vi "Can接收.vi"(7 "CANPort":u16, 9 "匹配CANID":u32 format="%x") -> (0 "接收数据":u8[](array[numeric]), 2 "成功？":bool)   [LabVIEW 2010]
uses:
  全局量/全局_配置.vi
panel:
  out "开始时间":dbl format="%#.0f"
  in  "Baudrate":u32(ring)=1000 caption="K" items=["10"=10, "20"=20, "50"=50, "100"=100, "125"=125, "250"=250, "500"=500, "800"=800, "250"=1000]
  out "Error out":errorcluster {"code" format="%.0x"}
  in  "ReadTimeOut":u32=3000 caption="ms"
  in  "Synchronization":i32(ring)=1 items=["Synchronization"=1, "Asynchronization"=0]
  # "从1开始"
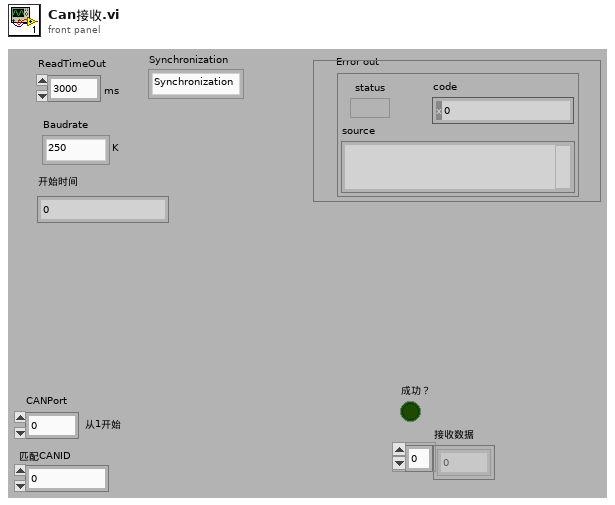
[diagram p1: front panel]
types:
  T1 = cluster{"Internal":u32, "InternalHigh":u32, "Offset":u32, "OffsetHigh":u32, "hEvent":u32}
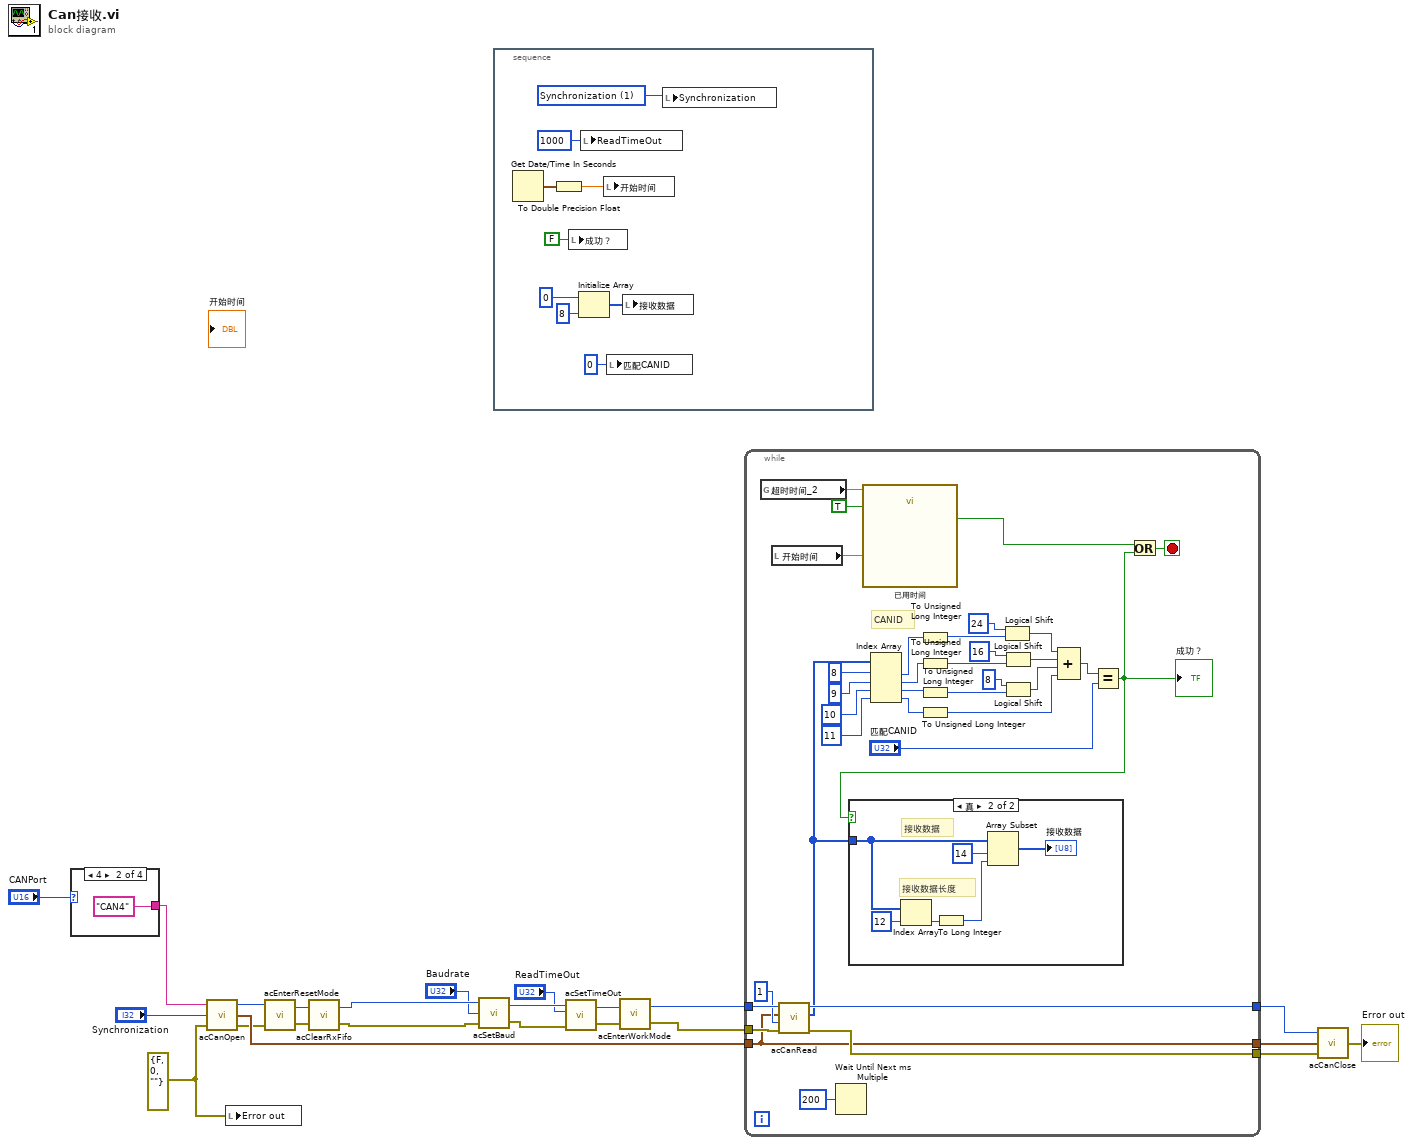
[diagram p0: block diagram]
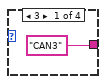
[diagram p3: hidden frame]
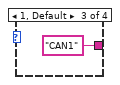
[diagram p4: hidden frame]
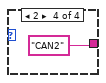
[diagram p5: hidden frame]
diagram:
  w17 = errorcluster {"status"=FALSE, "code"=0, "source"=""} ("Error in")
  n1 = case shown="4" "CANPort" {
    tunnel: ["CAN3" "CAN4" "CAN1" "CAN2"] -> w2
    frame 3 {
    }
    frame 4 {
    }
    frame 1, Default {
    }
    frame 2 {
    }
  }
  n2 = call "acCanOpen.vi"("Error in"=w17, "Synchronization"="Synchronization", "CANPort"=w2) -> ("Error out"=w18:errorcluster, "Overlapped"=w21:T1, "Handle"=w19:u32)
  n3 = local write "Error out"(w17) -> ()
  n4 = call "acEnterResetMode.vi"("Error in"=w18, "Handle  in"=w19) -> ("Error out"=w12:errorcluster, "Handle out"=w11:u32)
  n5 = call "acClearRxFifo.vi"("Error in"=w12, "Handle  in"=w11) -> ("Error out"=w9:errorcluster, "Handle out"=w10:u32)
  n6 = call "acSetBaud.vi"("Error in"=w9, "Baudrate"="Baudrate", "Handle  in"=w10) -> ("Error out"=w14:errorcluster, "Handle out"=w15:u32)
  n7 = stacked-sequence {
    frame #0 {
      w34 = 1 items=["Synchronization"=1, "Asynchronization"=0] ("Synchronization")
      n8 = Get Date/Time In Seconds() -> (seconds since 1Jan1904=w30:timestamp)
      n9 = To Double Precision Float(number=w30) -> (double precision float=w29:dbl)
      n10 = local write "成功？"(FALSE ("成功？")) -> ()
      n11 = Initialize Array(u8 0, 8 ("维数大小")) -> (w31:u8[])
      n12 = local write "ReadTimeOut"(u32 1000 ("ReadTimeOut")) -> ()
      n13 = local write "开始时间"(w29) -> ()
      n14 = local write "匹配CANID"(u32 0 ("匹配CANID")) -> ()
      n15 = local write "接收数据"(w31) -> ()
      n16 = local write "Synchronization"(w34) -> ()
    }
  }
  n17 = call "acSetTimeOut.vi"("Error in"=w14, "Read TimeOut"="ReadTimeOut", "Handle  in"=w15) -> ("Error out"=w7:errorcluster, "Handle out"=w8:u32)  [unwired: 1 in]
  n18 = call "acEnterWorkMode.vi"("Error in"=w7, "Handle  in"=w8) -> ("Error out"=w5:errorcluster, "Handle out"=w6:u32)
  n19 = while {
    tunnel: [w70] -> w22
    tunnel: w21 -> [w65]
    tunnel: [w69] -> w20
    tunnel: w6 -> [w68]
    tunnel: w5 -> [w67]
    tunnel: [w65] -> w1
    stop <- w60 stop-if-true
    # "CANID"
    n20 = global read "全局_配置.vi" "超时时间_2"() -> (w63:dbl)
    n21 = local read "开始时间"() -> (w62:dbl)
    n22 = call "acCanRead.vi"("Error in"=w67, "ReadCount"=u32 1 ("接收CAN帧数 2"), "Overlapped"=w65, "Handle  in"=w68) -> ("Error out"=w69:errorcluster, "MSG"=w38:u8[], "Handle out"=w70:u32)  [unwired: 1 out]
    n23 = Wait Until Next ms Multiple(millisecond multiple=u32 200 ("毫秒倍数")) -> ()  [unwired: 1 out]
    n24 = call "已用时间"("Time Target (s)"=w63, "Reset"=TRUE, "Set Start Time (s)"=w62) -> ("Time has Elapsed"=w61:bool)  [unwired: 9 in, 7 out]
    n25 = Index Array(array=w38, index #1=8 ("索引"), index #2=9 ("索引"), index #3=10 ("索引"), index #4=11 ("索引")) -> (element #1=w45:u8, element #2=w44:u8, element #3=w41:u8, element #4=w40:u8)
    n26 = To Unsigned Long Integer(number=w45) -> (unsigned 32bit integer=w46:u32)
    n27 = To Unsigned Long Integer(number=w44) -> (unsigned 32bit integer=w43:u32)
    n28 = To Unsigned Long Integer(number=w41) -> (unsigned 32bit integer=w42:u32)
    n29 = To Unsigned Long Integer(number=w40) -> (unsigned 32bit integer=w39:u32)
    n30 = Logical Shift(y=i8 24, x=w46) -> (x << y=w50:u32)
    n31 = Logical Shift(y=i8 16, x=w43) -> (x << y=w51:u32)
    n32 = Logical Shift(y=i8 8, x=w42) -> (x << y=w49:u32)
    n33 = Compound Arithmetic op=ADD(w50, w51, w49, w39) -> (w48:u32)
    n34 = Equal?(x=w48, y="匹配CANID") -> (x = y?=w37:bool)
    "成功？" <- w37
    n35 = case shown="真" w37 {
      tunnel: w38 -> [_ w71]
      frame False {
      }
      frame True {
        # "接收数据"
        # "接收数据长度"
        n36 = Index Array(array=w71, index=12 ("索引")) -> (element=w74:u8)
        n37 = To Long Integer(number=w74) -> (32bit integer=w73:i32)
        n38 = Array Subset(array=w71, index=14 ("索引"), length=w73) -> (→"接收数据":u8[])
      }
    }
    n39 = Or(x=w61, y=w37) -> (x .or. y?=w60:bool)
  }
  n40 = call "acCanClose.vi"("Error in"=w20, "Overlapped"=w1, "Handle  in"=w22) -> ("Error out"=→"Error out":errorcluster)
